vi "Slave - Latency Bmk.vi"() -> ()   [LabVIEW 2016]
uses:
  <vilib>/Utility/error.llb/DialogType.ctl
  <vilib>/Analysis/baseanly.llb/Mean (DBL).vi
  <vilib>/pximc/Initialize Writer Session (DBL).vi
  <vilib>/pximc/Initialize Reader Session (DBL).vi
  <vilib>/pximc/Connect (DBL).vi
  <vilib>/pximc/Write (DBL).vi
  <vilib>/pximc/Read (DBL).vi
  <vilib>/pximc/nipximc.lvlib
  <vilib>/Analysis/NI_AALBase.lvlib
panel:
  out "N1=>N2 Received vs Generated Samples Ratio (%)":dbl
  out "N2=>N1 Received vs Generated Samples Ratio (%)":dbl
  out "Avg Latency":dbl
  out "N2=>N1 Avg Latency":dbl
  out "Value Change Timestamp 2":u32 caption="Tick Count(uSec)"
  out "N1=>N2 Avg Latency":dbl
  out "Value Change Timestamp":u32 caption="Tick Count(uSec)"
  in  "Node 1 Reader Connection ID":u16=4
  in  "Reader Interface Node 2":tag="PXIMC2" caption="interface"
  in  "Node 2 Writer Connection ID":u16=3
  in  "Writer Interface Node 2":tag="PXIMC2" caption="interface"
  out "Stopped?":bool
  in  "Node 1 Writer Connection ID":u16=1
  in  "Node 1 Writer Interface":tag="PXIMC2" caption="interface"
  in  "Stop Button":bool
  in  "Node 1 Reader Interface":tag="PXIMC2" caption="interface"
  in  "Buffer Size":u64=250000 caption="buffer size"
  in  "Connection Timeout (s)":dbl=60.0 caption="timeout in seconds (-1)"
  in  "Node 1 Reader Connection ID":u16=2
  # "Node 1"
  # "Node 2"
  # "Node 2 => Node 1"
  # "Node 1 => Node 2"
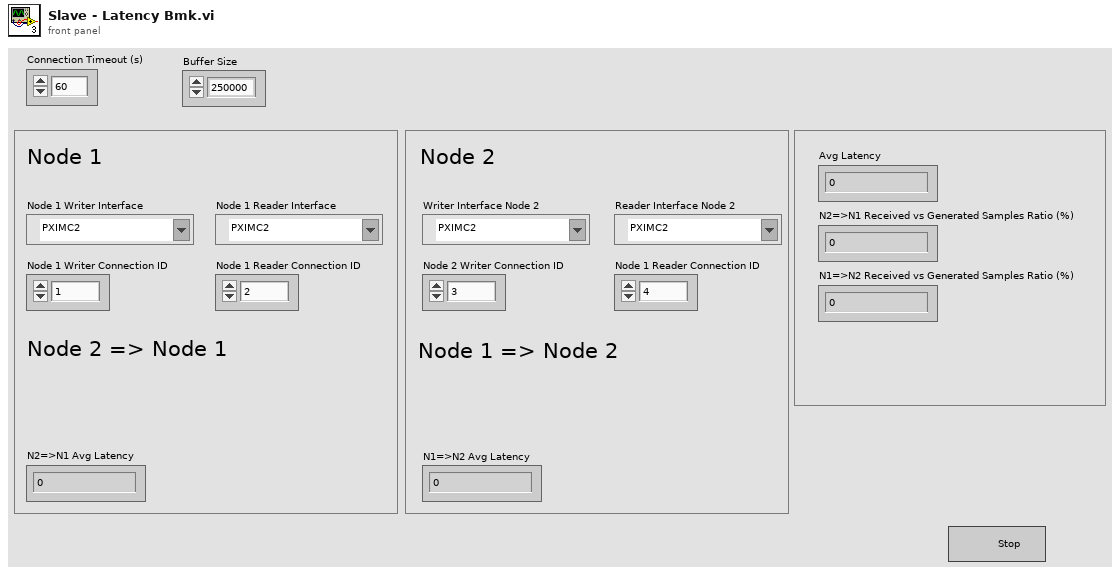
[diagram p1: front panel]
types:
  T1 = typedef "DialogType.ctl" = u16
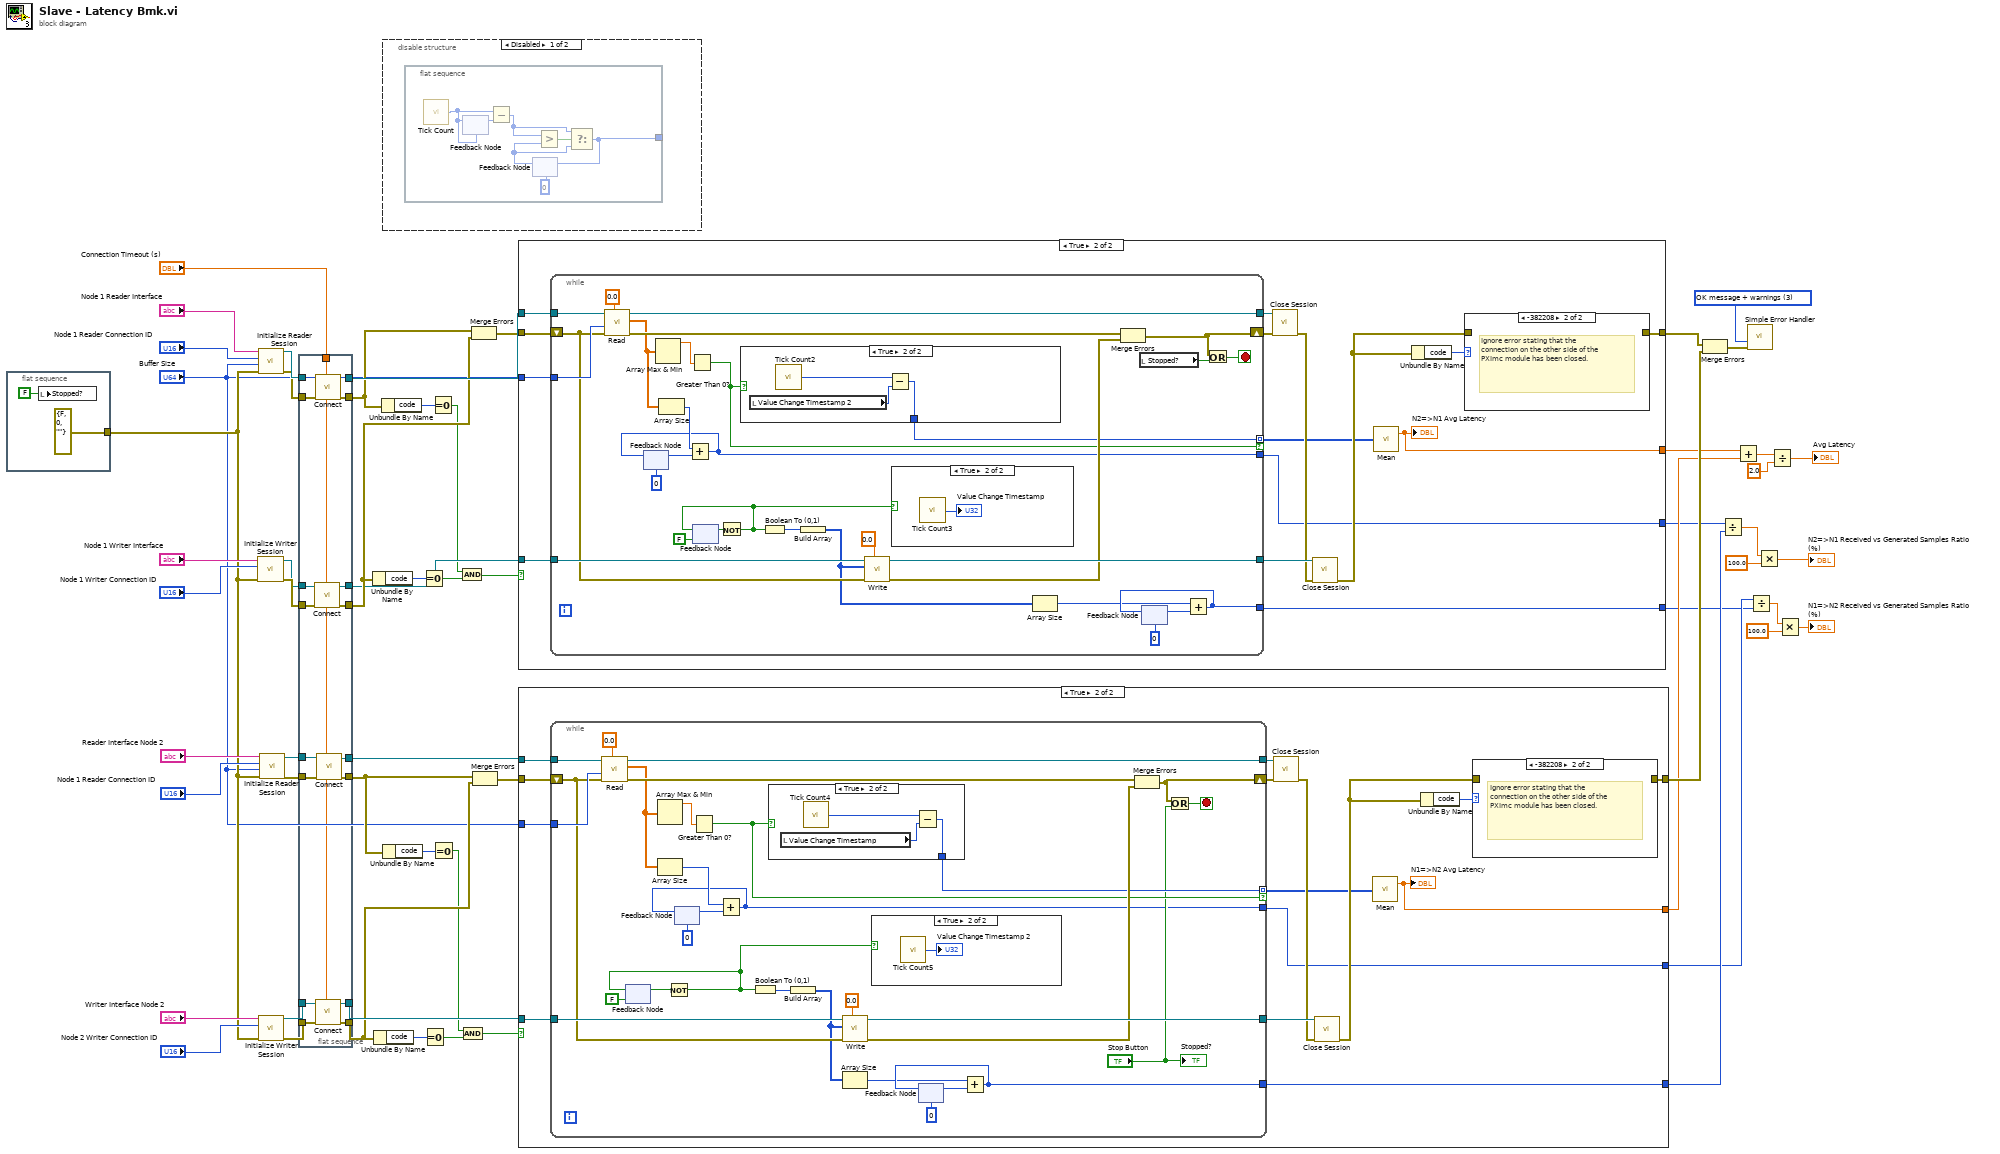
[diagram p0: block diagram]
diagram:
  w52 = T1 3 items=["no dialog", "OK message", "continue or stop message", "OK message + warnings", "continue/stop + warnings"] ("type of dialog (OK msg:1)")
  n1 = flat-sequence {
    tunnel: [errorcluster {"status"=FALSE, "code"=0, "source"=""} ("error constant")] -> w21
    frame #0 {
      n2 = local write "Stopped?"(FALSE ("Stopped?")) -> ()
    }
  }
  n3 = call-poly <vilib>:"Initialize Writer Session.vi"("error in (no error)"=w21, "connection id (1)"="Node 1 Writer Connection ID", "interface"="Node 1 Writer Interface") -> ("error out"=w50:errorcluster, "session out"=w49:refnum<k21>)  [unwired: 7 in]
  n4 = call-poly <vilib>:"Initialize Reader Session.vi"("error in (no error)"=w21, "buffer size"="Buffer Size", "writer's connection id (1)"="Node 1 Reader Connection ID", "interface"="Node 1 Reader Interface") -> ("error out"=w56:errorcluster, "session out"=w57:refnum<k21>)  [unwired: 6 in]
  n5 = call-poly <vilib>:"Initialize Writer Session.vi"("error in (no error)"=w21, "connection id (1)"="Node 2 Writer Connection ID", "interface"="Writer Interface Node 2") -> ("error out"=w29:errorcluster, "session out"=w30:refnum<k21>)  [unwired: 7 in]
  n6 = call-poly <vilib>:"Initialize Reader Session.vi"("error in (no error)"=w21, "buffer size"="Buffer Size", "writer's connection id (1)"="Node 1 Reader Connection ID", "interface"="Reader Interface Node 2") -> ("error out"=w24:errorcluster, "session out"=w23:refnum<k21>)  [unwired: 6 in]
  n7 = flat-sequence {
    tunnel: w57 -> [w77]
    tunnel: w56 -> [w76]
    tunnel: [w75] -> w55
    tunnel: w50 -> [w74]
    tunnel: w49 -> [w73]
    tunnel: [w72] -> w43
    tunnel: [w71] -> w42
    tunnel: "Connection Timeout (s)" -> [w61]
    tunnel: [w70] -> w40
    tunnel: [w69] -> w39
    tunnel: [w68] -> w38
    tunnel: [w67] -> w37
    tunnel: w30 -> [w66]
    tunnel: w29 -> [w65]
    tunnel: [w64] -> w25
    tunnel: w24 -> [w63]
    tunnel: w23 -> [w62]
    frame #0 {
      n8 = call-poly <vilib>:"Connect.vi"("timeout in seconds (-1)"=w61, "error in (no error)"=w74, "session in"=w73) -> ("error out"=w71:errorcluster, "session out"=w70:refnum<k21>)  [unwired: 7 in]
      n9 = call-poly <vilib>:"Connect.vi"("timeout in seconds (-1)"=w61, "error in (no error)"=w76, "session in"=w77) -> ("error out"=w72:errorcluster, "session out"=w75:refnum<k21>)  [unwired: 7 in]
      n10 = call-poly <vilib>:"Connect.vi"("timeout in seconds (-1)"=w61, "error in (no error)"=w65, "session in"=w66) -> ("error out"=w68:errorcluster, "session out"=w69:refnum<k21>)  [unwired: 7 in]
      n11 = call-poly <vilib>:"Connect.vi"("timeout in seconds (-1)"=w61, "error in (no error)"=w63, "session in"=w62) -> ("error out"=w67:errorcluster, "session out"=w64:refnum<k21>)  [unwired: 7 in]
    }
  }
  n12 = Unbundle By Name(w42) -> ("code"=w47:i32)
  n13 = Unbundle By Name(w38) -> ("code"=w32:i32)
  n14 = Unbundle By Name(w43) -> ("code"=w53:i32)
  n15 = disable-structure shown="Disabled" {
    frame Disabled {
      n16 = flat-sequence {
        tunnel: [w78] -> _
        frame #0 {
          n17 = call "Tick Count"() -> ("Tick Count(uSec)"=w79:u32)
          n18 = feedback #1(w79) -> (w83:u32)
          n19 = feedback-in #1(w79) -> ()
          n20 = Subtract(x=w79, y=w83) -> (x-y=w84:u32)
          n21 = feedback #2(u32 0) -> (w80:u32)
          n22 = Greater?(x=w84, y=w80) -> (0:w81:bool)
          n23 = Select(t=w84, s=w81, f=w80) -> (s? t:f=w78:u32)
          n24 = feedback-in #2(w78) -> ()
        }
      }
    }
    frame Enabled {
    }
  }
  n25 = Unbundle By Name(w37) -> ("code"=w27:i32)
  n26 = Equal To 0?(x=w47) -> (x = 0?=w45:bool)
  n27 = Equal To 0?(x=w32) -> (x = 0?=w35:bool)
  n28 = Equal To 0?(x=w53) -> (x = 0?=w19:bool)
  n29 = Equal To 0?(x=w27) -> (x = 0?=w34:bool)
  n30 = And(x=w19, y=w45) -> (x .and. y?=w46:bool)
  n31 = And(x=w34, y=w35) -> (x .and. y?=w33:bool)
  n32 = Merge Errors(w43, w42) -> (w44:errorcluster)
  n33 = Merge Errors(w37, w38) -> (w36:errorcluster)
  n34 = case shown="True" w46 {
    tunnel: w44 -> [w85 w100]
    tunnel: w55 -> [_ w99]
    tunnel: [w85 w97] -> w18
    tunnel: "Buffer Size" -> [_ w94]
    tunnel: w40 -> [_ w93]
    tunnel: [_ w88] -> w14
    tunnel: [_ w87] -> w10
    tunnel: [_ w86] -> w1
    frame False {
      # "The connection was not successful for some reason."
    }
    frame True {
      n35 = while {
        tunnel: w99 -> [w130]
        tunnel: [w129] -> w98
        shift-right: [w122] -> w95
        shift-left: w100 -> [w116]
        tunnel: w94 -> [w128]
        tunnel: w93 -> [w127]
        tunnel: [w126] -> w92
        tunnel: [w114] -> w89 mode=indexing if=w113
        tunnel: [w108] -> w86
        tunnel: [w103] -> w87
        stop <- w123 stop-if-true
        n36 = call-poly <vilib>:"Read.vi"("timeout in seconds (5)"=0.0, "error in (no error)"=w116, "number of elements"=w128, "session in"=w130) -> ("error out"=w125:errorcluster, "data"=w105:dbl[], "session out"=w129:refnum<k21>)  [unwired: 5 in]
        n37 = feedback #3(0) -> (w106:i32)
        n38 = Array Max & Min(array=w105) -> (max value=w115:dbl)  [unwired: 3 out]
        n39 = Array Size(array=w105) -> (size(s)=w104:i32)
        n40 = Add(x=w104, y=w106) -> (x+y=w103:i32)
        n41 = feedback-in #3(w103) -> ()
        n42 = Greater Than 0?(x=w115) -> (x > 0?=w113:bool)
        n43 = feedback #4(FALSE) -> (w118:bool)
        n44 = Not(x=w118) -> (.not. x?=w117:bool)
        n45 = feedback-in #4(w117) -> ()
        n46 = case shown="True" w113 {
          tunnel: [_ w131] -> w114
          frame False {
          }
          frame True {
            n47 = local read "Value Change Timestamp 2"() -> (w133:u32)
            n48 = call "Tick Count2"() -> ("Tick Count(uSec)"=w132:u32)
            n49 = Subtract(x=w132, y=w133) -> (x-y=w131:u32)
          }
        }
        n50 = Boolean To (0,1)(Boolean=w117) -> (0, 1=w109:i16)
        n51 = Build Array(w109) -> (w102:i16[])
        n52 = call-poly <vilib>:"Write.vi"("timeout in seconds (5)"=0.0, "error in (no error)"=w116, "data"=w102, "session in"=w127) -> ("error out"=w124:errorcluster, "session out"=w126:refnum<k21>)  [unwired: 5 in, 1 out]
        n53 = case shown="True" w117 {
          frame False {
          }
          frame True {
            n54 = call "Tick Count3"() -> ("Tick Count(uSec)"=→"Value Change Timestamp":u32)
          }
        }
        n55 = Array Size(array=w102) -> (size(s)=w101:i32)
        n56 = Merge Errors(w125, w124) -> (w122:errorcluster)
        n57 = local read "Stopped?"() -> (w112:bool)
        n58 = feedback #5(0) -> (w111:i32)
        n59 = Add(x=w101, y=w111) -> (x+y=w108:i32)
        n60 = feedback-in #5(w108) -> ()
        n61 = Or(x=w122, y=w112) -> (x .or. y?=w123:bool)
      }
      n62 = call <vilib>:"Close Session.vi"("error in (no error)"=w95, "session in"=w98) -> ("error out"=w91:errorcluster)  [unwired: 9 in]
      n63 = call <vilib>:"Close Session.vi"("error in (no error)"=w91, "session in"=w92) -> ("error out"=w90:errorcluster)  [unwired: 9 in]
      n64 = call-poly <vilib>:"Mean.vi"("X"=w89) -> ("mean"=w88:dbl)  [unwired: 1 out]
      "N2=>N1 Avg Latency" <- w88
      n65 = Unbundle By Name(w90) -> ("code"=w96:i32)
      n66 = case shown="-382208" w96 {
        tunnel: w90 -> [w135 _]
        tunnel: [w135 _] -> w97
        frame 0, Default {
        }
        frame -382208 {
          # "Ignore error stating that the connection on the other side of the PXImc module has been closed."
        }
      }
    }
  }
  n67 = case shown="True" w33 {
    tunnel: w36 -> [w136 w151]
    tunnel: w25 -> [_ w150]
    tunnel: [w136 w148] -> w17
    tunnel: "Buffer Size" -> [_ w145]
    tunnel: w39 -> [_ w144]
    tunnel: [_ w139] -> w13
    tunnel: [_ w138] -> w2
    tunnel: [_ w137] -> w9
    frame False {
      # "The connection was not successful for some reason."
    }
    frame True {
      n68 = while {
        tunnel: w150 -> [w181]
        tunnel: [w180] -> w149
        shift-right: [w173] -> w146
        shift-left: w151 -> [w167]
        tunnel: w145 -> [w179]
        tunnel: w144 -> [w178]
        tunnel: [w177] -> w143
        tunnel: [w170] -> w140 mode=indexing if=w169
        tunnel: [w158] -> w138
        tunnel: [w154] -> w137
        stop <- w174 stop-if-true
        n69 = call-poly <vilib>:"Read.vi"("timeout in seconds (5)"=0.0, "error in (no error)"=w167, "number of elements"=w179, "session in"=w181) -> ("error out"=w176:errorcluster, "data"=w162:dbl[], "session out"=w180:refnum<k21>)  [unwired: 5 in]
        n70 = feedback #6(FALSE) -> (w164:bool)
        n71 = Array Max & Min(array=w162) -> (max value=w166:dbl)  [unwired: 3 out]
        n72 = Array Size(array=w162) -> (size(s)=w160:i32)
        n73 = Not(x=w164) -> (.not. x?=w163:bool)
        n74 = feedback-in #6(w163) -> ()
        n75 = feedback #7(0) -> (w159:i32)
        n76 = Greater Than 0?(x=w166) -> (x > 0?=w169:bool)
        n77 = Add(x=w160, y=w159) -> (x+y=w158:i32)
        n78 = feedback-in #7(w158) -> ()
        n79 = Boolean To (0,1)(Boolean=w163) -> (0, 1=w155:i16)
        n80 = case shown="True" w169 {
          tunnel: [_ w183] -> w170
          frame False {
          }
          frame True {
            n81 = local read "Value Change Timestamp"() -> (w185:u32)
            n82 = call "Tick Count4"() -> ("Tick Count(uSec)"=w184:u32)
            n83 = Subtract(x=w184, y=w185) -> (x-y=w183:u32)
          }
        }
        n84 = Build Array(w155) -> (w153:i16[])
        n85 = call-poly <vilib>:"Write.vi"("timeout in seconds (5)"=0.0, "error in (no error)"=w167, "data"=w153, "session in"=w178) -> ("error out"=w175:errorcluster, "session out"=w177:refnum<k21>)  [unwired: 5 in, 1 out]
        n86 = Array Size(array=w153) -> (size(s)=w152:i32)
        n87 = case shown="True" w163 {
          frame False {
          }
          frame True {
            n88 = call "Tick Count5"() -> ("Tick Count(uSec)"=→"Value Change Timestamp 2":u32)
          }
        }
        n89 = feedback #8(0) -> (w156:i32)
        n90 = Add(x=w152, y=w156) -> (x+y=w154:i32)
        n91 = feedback-in #8(w154) -> ()
        n92 = Merge Errors(w176, w175) -> (w173:errorcluster)
        n93 = Or(x=w173, y="Stop Button") -> (x .or. y?=w174:bool)
        "Stopped?" <- "Stop Button"
      }
      n94 = call <vilib>:"Close Session.vi"("error in (no error)"=w146, "session in"=w149) -> ("error out"=w142:errorcluster)  [unwired: 9 in]
      n95 = call <vilib>:"Close Session.vi"("error in (no error)"=w142, "session in"=w143) -> ("error out"=w141:errorcluster)  [unwired: 9 in]
      n96 = call-poly <vilib>:"Mean.vi"("X"=w140) -> ("mean"=w139:dbl)  [unwired: 1 out]
      "N1=>N2 Avg Latency" <- w139
      n97 = Unbundle By Name(w141) -> ("code"=w147:i32)
      n98 = case shown="-382208" w147 {
        tunnel: w141 -> [w186 _]
        tunnel: [w186 _] -> w148
        frame 0, Default {
        }
        frame -382208 {
          # "Ignore error stating that the connection on the other side of the PXImc module has been closed."
        }
      }
    }
  }
  n99 = Merge Errors(w18, w17) -> (w16:errorcluster)
  n100 = Divide(x=w10, y=w9) -> (x/y=w8:dbl)
  n101 = Add(x=w14, y=w13) -> (x+y=w15:dbl)
  n102 = call <vilib>:"Simple Error Handler.vi"("type of dialog (OK msg:1)"=w52, "error in (no error)"=w16) -> ()  [unwired: 3 in, 5 out]
  n103 = Divide(x=w2, y=w1) -> (x/y=w4:dbl)
  n104 = Multiply(x=w8, y=100.0) -> (x*y=→"N2=>N1 Received vs Generated Samples Ratio (%)":dbl)
  n105 = Divide(x=w15, y=2.0) -> (x/y=→"Avg Latency":dbl)
  n106 = Multiply(x=w4, y=100.0) -> (x*y=→"N1=>N2 Received vs Generated Samples Ratio (%)":dbl)
